vi "Call Scan Code.vi"(0 "timeout (10sec)":u32=10000 caption="超时（10秒）", 1 "baud rate (9600)":u32=9600 caption="波特率(9600)", 2 "data bits (8)":u16=8 caption="数据比特(8)" min=5 max=8 step=1, 3 "parity (0:none)":enum16{"None", "Odd", "Even", "Mark", "Space"}(ring) caption="奇偶（0:无）", 4 "写入缓冲区":string, 5 "Total Bytes":u32, 6 "Station 1":refnum<visa-resource-name>, 7 "Station 4":refnum<visa-resource-name>, 8 "Station 2":refnum<visa-resource-name>, 9 "Station 5":refnum<visa-resource-name>, 10 "Station 3":refnum<visa-resource-name>, 11 "Station 6":refnum<visa-resource-name>) -> (14 "Station 1 data":string, 15 "Station 2 data":string, 16 "Station 3 data":string, 17 "Station 4 data":string, 18 "Station 5 data":string, 19 "Station 6 data":string)   [LabVIEW 2014]
uses:
  <vilib>/Instr/_visa.llb/VISA Configure Serial Port (Instr).vi
panel:
  out "Error 6":errorcluster caption="错误输出"
  out "Error 5":errorcluster caption="错误输出"
  out "Error 4":errorcluster caption="错误输出"
  out "Error 3":errorcluster caption="错误输出"
  out "Error 2":errorcluster caption="错误输出"
  out "Error":errorcluster caption="错误输出"
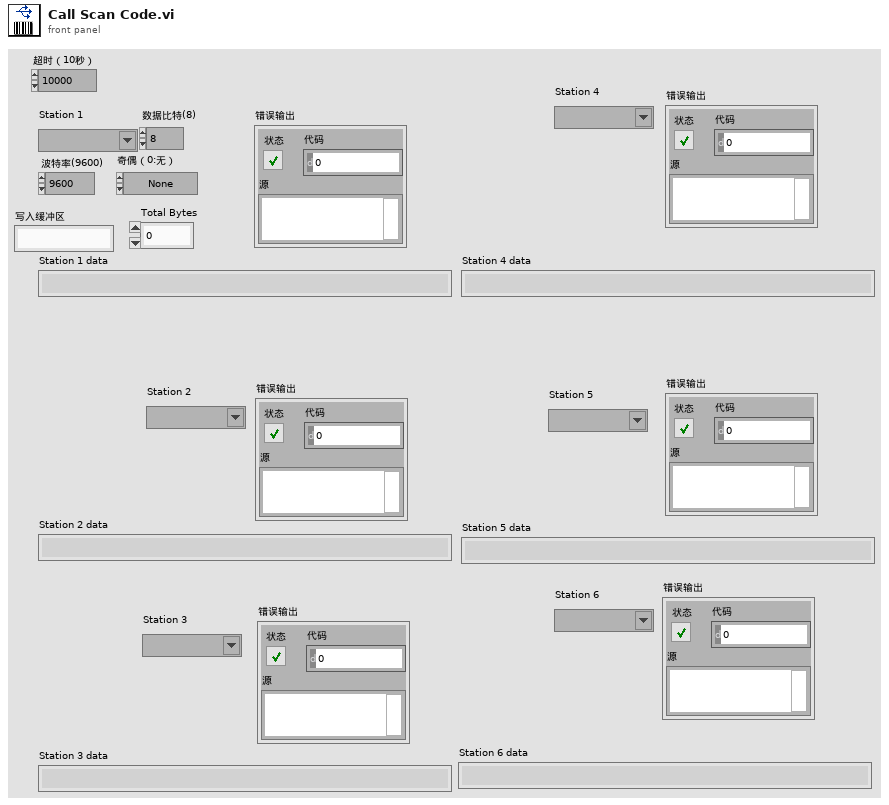
[diagram p1: front panel]
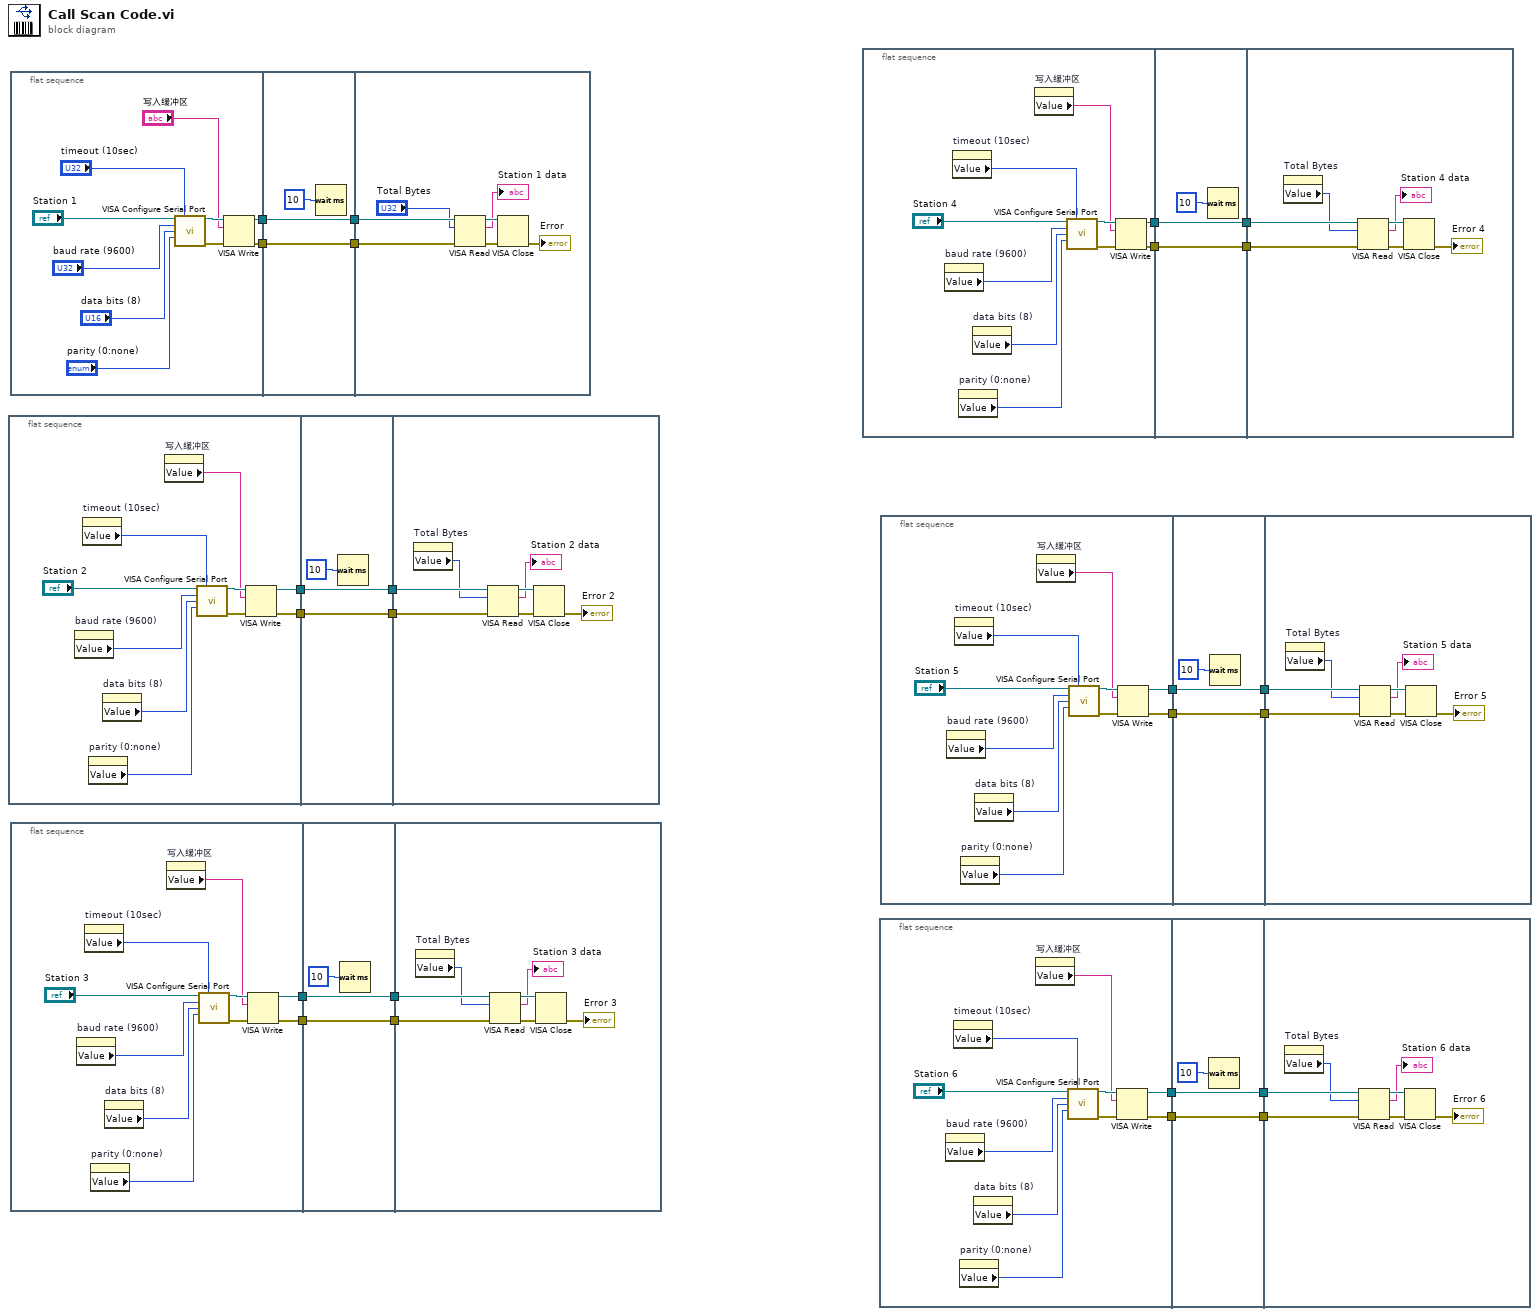
[diagram p0: block diagram]
diagram:
  n1 = flat-sequence {
    tunnel: [w31] -> w20
    tunnel: [w30] -> w19
    tunnel: [w36] -> w18
    tunnel: w20 -> [w36]
    tunnel: [w35] -> w17
    tunnel: w19 -> [w35]
    tunnel: w18 -> [w44]
    tunnel: w17 -> [w43]
    frame #0 {
      n2 = property on="baud rate (9600)" class="DigNum (严格)"() -> ("Value"=w28:u32)  [unwired: 2 in, 2 out]
      n3 = property on="timeout (10sec)" class="DigNum (严格)"() -> ("Value"=w29:u32)  [unwired: 2 in, 2 out]
      n4 = property on="parity (0:none)" class="Enum (严格)"() -> ("Value"=w26:enum16{"None", "Odd", "Even", "Mark", "Space"})  [unwired: 2 in, 2 out]
      n5 = property on="data bits (8)" class="DigNum (严格)"() -> ("Value"=w27:u16)  [unwired: 2 in, 2 out]
      n6 = property on="写入缓冲区" class="Str"() -> ("Value"=w25:string)  [unwired: 2 in, 2 out]
      n7 = call-poly "VISA Configure Serial Port"("VISA resource name"="Station 2", "timeout (10sec)"=w29, "baud rate (9600)"=w28, "data bits (8)"=w27, "parity (0:none)"=w26) -> ("VISA resource name out"=w33:refnum<visa-resource-name>, "error out"=w32:errorcluster)  [unwired: 9 in]
      n8 = VISA Write(VISA resource name=w33, write buffer=w25, error in (no error)=w32) -> (VISA resource name out=w31:refnum<visa-resource-name>, error out=w30:errorcluster)  [unwired: 1 out]
    }
    frame #1 {
      n9 = Wait (ms)(milliseconds to wait=u32 10 ("等待时间（毫秒）")) -> ()  [unwired: 1 out]
    }
    frame #2 {
      n10 = property on="Total Bytes" class="DigNum (严格)"() -> ("Value"=w38:u32)  [unwired: 2 in, 2 out]
      n11 = VISA Read(VISA resource name=w44, byte count=w38, error in (no error)=w43) -> (VISA resource name out=w42:refnum<visa-resource-name>, read buffer=→"Station 2 data":string, error out=w41:errorcluster)  [unwired: 1 out]
      n12 = VISA Close(VISA resource name=w42, error in (no error)=w41) -> (error out=→"Error 2":errorcluster)
    }
  }
  n13 = flat-sequence {
    tunnel: [w48] -> w24
    tunnel: [w47] -> w23
    tunnel: [w56] -> w22
    tunnel: w24 -> [w56]
    tunnel: [w55] -> w21
    tunnel: w23 -> [w55]
    tunnel: w22 -> [w64]
    tunnel: w21 -> [w63]
    frame #0 {
      n14 = call-poly "VISA Configure Serial Port"("VISA resource name"="Station 1", "timeout (10sec)"="timeout (10sec)", "baud rate (9600)"="baud rate (9600)", "data bits (8)"="data bits (8)", "parity (0:none)"="parity (0:none)") -> ("VISA resource name out"=w50:refnum<visa-resource-name>, "error out"=w49:errorcluster)  [unwired: 9 in]
      n15 = VISA Write(VISA resource name=w50, write buffer="写入缓冲区", error in (no error)=w49) -> (VISA resource name out=w48:refnum<visa-resource-name>, error out=w47:errorcluster)  [unwired: 1 out]
    }
    frame #1 {
      n16 = Wait (ms)(milliseconds to wait=u32 10 ("等待时间（毫秒）")) -> ()  [unwired: 1 out]
    }
    frame #2 {
      n17 = VISA Read(VISA resource name=w64, byte count="Total Bytes", error in (no error)=w63) -> (VISA resource name out=w61:refnum<visa-resource-name>, read buffer=→"Station 1 data":string, error out=w60:errorcluster)  [unwired: 1 out]
      n18 = VISA Close(VISA resource name=w61, error in (no error)=w60) -> (error out=→"Error":errorcluster)
    }
  }
  n19 = flat-sequence {
    tunnel: [w71] -> w16
    tunnel: [w70] -> w15
    tunnel: [w76] -> w14
    tunnel: w16 -> [w76]
    tunnel: [w75] -> w13
    tunnel: w15 -> [w75]
    tunnel: w14 -> [w84]
    tunnel: w13 -> [w83]
    frame #0 {
      n20 = property on="baud rate (9600)" class="DigNum (严格)"() -> ("Value"=w68:u32)  [unwired: 2 in, 2 out]
      n21 = property on="timeout (10sec)" class="DigNum (严格)"() -> ("Value"=w69:u32)  [unwired: 2 in, 2 out]
      n22 = property on="parity (0:none)" class="Enum (严格)"() -> ("Value"=w66:enum16{"None", "Odd", "Even", "Mark", "Space"})  [unwired: 2 in, 2 out]
      n23 = property on="data bits (8)" class="DigNum (严格)"() -> ("Value"=w67:u16)  [unwired: 2 in, 2 out]
      n24 = property on="写入缓冲区" class="Str"() -> ("Value"=w65:string)  [unwired: 2 in, 2 out]
      n25 = call-poly "VISA Configure Serial Port"("VISA resource name"="Station 3", "timeout (10sec)"=w69, "baud rate (9600)"=w68, "data bits (8)"=w67, "parity (0:none)"=w66) -> ("VISA resource name out"=w73:refnum<visa-resource-name>, "error out"=w72:errorcluster)  [unwired: 9 in]
      n26 = VISA Write(VISA resource name=w73, write buffer=w65, error in (no error)=w72) -> (VISA resource name out=w71:refnum<visa-resource-name>, error out=w70:errorcluster)  [unwired: 1 out]
    }
    frame #1 {
      n27 = Wait (ms)(milliseconds to wait=u32 10 ("等待时间（毫秒）")) -> ()  [unwired: 1 out]
    }
    frame #2 {
      n28 = property on="Total Bytes" class="DigNum (严格)"() -> ("Value"=w78:u32)  [unwired: 2 in, 2 out]
      n29 = VISA Read(VISA resource name=w84, byte count=w78, error in (no error)=w83) -> (VISA resource name out=w82:refnum<visa-resource-name>, read buffer=→"Station 3 data":string, error out=w81:errorcluster)  [unwired: 1 out]
      n30 = VISA Close(VISA resource name=w82, error in (no error)=w81) -> (error out=→"Error 3":errorcluster)
    }
  }
  n31 = flat-sequence {
    tunnel: [w91] -> w12
    tunnel: [w90] -> w11
    tunnel: [w96] -> w10
    tunnel: w12 -> [w96]
    tunnel: [w95] -> w9
    tunnel: w11 -> [w95]
    tunnel: w10 -> [w104]
    tunnel: w9 -> [w103]
    frame #0 {
      n32 = property on="baud rate (9600)" class="DigNum (严格)"() -> ("Value"=w88:u32)  [unwired: 2 in, 2 out]
      n33 = property on="timeout (10sec)" class="DigNum (严格)"() -> ("Value"=w89:u32)  [unwired: 2 in, 2 out]
      n34 = property on="parity (0:none)" class="Enum (严格)"() -> ("Value"=w86:enum16{"None", "Odd", "Even", "Mark", "Space"})  [unwired: 2 in, 2 out]
      n35 = property on="data bits (8)" class="DigNum (严格)"() -> ("Value"=w87:u16)  [unwired: 2 in, 2 out]
      n36 = property on="写入缓冲区" class="Str"() -> ("Value"=w85:string)  [unwired: 2 in, 2 out]
      n37 = call-poly "VISA Configure Serial Port"("VISA resource name"="Station 4", "timeout (10sec)"=w89, "baud rate (9600)"=w88, "data bits (8)"=w87, "parity (0:none)"=w86) -> ("VISA resource name out"=w93:refnum<visa-resource-name>, "error out"=w92:errorcluster)  [unwired: 9 in]
      n38 = VISA Write(VISA resource name=w93, write buffer=w85, error in (no error)=w92) -> (VISA resource name out=w91:refnum<visa-resource-name>, error out=w90:errorcluster)  [unwired: 1 out]
    }
    frame #1 {
      n39 = Wait (ms)(milliseconds to wait=u32 10 ("等待时间（毫秒）")) -> ()  [unwired: 1 out]
    }
    frame #2 {
      n40 = property on="Total Bytes" class="DigNum (严格)"() -> ("Value"=w98:u32)  [unwired: 2 in, 2 out]
      n41 = VISA Read(VISA resource name=w104, byte count=w98, error in (no error)=w103) -> (VISA resource name out=w102:refnum<visa-resource-name>, read buffer=→"Station 4 data":string, error out=w101:errorcluster)  [unwired: 1 out]
      n42 = VISA Close(VISA resource name=w102, error in (no error)=w101) -> (error out=→"Error 4":errorcluster)
    }
  }
  n43 = flat-sequence {
    tunnel: [w111] -> w4
    tunnel: [w110] -> w3
    tunnel: [w116] -> w2
    tunnel: w4 -> [w116]
    tunnel: [w115] -> w1
    tunnel: w3 -> [w115]
    tunnel: w2 -> [w124]
    tunnel: w1 -> [w123]
    frame #0 {
      n44 = property on="baud rate (9600)" class="DigNum (严格)"() -> ("Value"=w108:u32)  [unwired: 2 in, 2 out]
      n45 = property on="timeout (10sec)" class="DigNum (严格)"() -> ("Value"=w109:u32)  [unwired: 2 in, 2 out]
      n46 = property on="parity (0:none)" class="Enum (严格)"() -> ("Value"=w106:enum16{"None", "Odd", "Even", "Mark", "Space"})  [unwired: 2 in, 2 out]
      n47 = property on="data bits (8)" class="DigNum (严格)"() -> ("Value"=w107:u16)  [unwired: 2 in, 2 out]
      n48 = property on="写入缓冲区" class="Str"() -> ("Value"=w105:string)  [unwired: 2 in, 2 out]
      n49 = call-poly "VISA Configure Serial Port"("VISA resource name"="Station 6", "timeout (10sec)"=w109, "baud rate (9600)"=w108, "data bits (8)"=w107, "parity (0:none)"=w106) -> ("VISA resource name out"=w113:refnum<visa-resource-name>, "error out"=w112:errorcluster)  [unwired: 9 in]
      n50 = VISA Write(VISA resource name=w113, write buffer=w105, error in (no error)=w112) -> (VISA resource name out=w111:refnum<visa-resource-name>, error out=w110:errorcluster)  [unwired: 1 out]
    }
    frame #1 {
      n51 = Wait (ms)(milliseconds to wait=u32 10 ("等待时间（毫秒）")) -> ()  [unwired: 1 out]
    }
    frame #2 {
      n52 = property on="Total Bytes" class="DigNum (严格)"() -> ("Value"=w118:u32)  [unwired: 2 in, 2 out]
      n53 = VISA Read(VISA resource name=w124, byte count=w118, error in (no error)=w123) -> (VISA resource name out=w122:refnum<visa-resource-name>, read buffer=→"Station 6 data":string, error out=w121:errorcluster)  [unwired: 1 out]
      n54 = VISA Close(VISA resource name=w122, error in (no error)=w121) -> (error out=→"Error 6":errorcluster)
    }
  }
  n55 = flat-sequence {
    tunnel: [w131] -> w8
    tunnel: [w130] -> w7
    tunnel: [w136] -> w6
    tunnel: w8 -> [w136]
    tunnel: [w135] -> w5
    tunnel: w7 -> [w135]
    tunnel: w6 -> [w144]
    tunnel: w5 -> [w143]
    frame #0 {
      n56 = property on="baud rate (9600)" class="DigNum (严格)"() -> ("Value"=w128:u32)  [unwired: 2 in, 2 out]
      n57 = property on="timeout (10sec)" class="DigNum (严格)"() -> ("Value"=w129:u32)  [unwired: 2 in, 2 out]
      n58 = property on="parity (0:none)" class="Enum (严格)"() -> ("Value"=w126:enum16{"None", "Odd", "Even", "Mark", "Space"})  [unwired: 2 in, 2 out]
      n59 = property on="data bits (8)" class="DigNum (严格)"() -> ("Value"=w127:u16)  [unwired: 2 in, 2 out]
      n60 = property on="写入缓冲区" class="Str"() -> ("Value"=w125:string)  [unwired: 2 in, 2 out]
      n61 = call-poly "VISA Configure Serial Port"("VISA resource name"="Station 5", "timeout (10sec)"=w129, "baud rate (9600)"=w128, "data bits (8)"=w127, "parity (0:none)"=w126) -> ("VISA resource name out"=w133:refnum<visa-resource-name>, "error out"=w132:errorcluster)  [unwired: 9 in]
      n62 = VISA Write(VISA resource name=w133, write buffer=w125, error in (no error)=w132) -> (VISA resource name out=w131:refnum<visa-resource-name>, error out=w130:errorcluster)  [unwired: 1 out]
    }
    frame #1 {
      n63 = Wait (ms)(milliseconds to wait=u32 10 ("等待时间（毫秒）")) -> ()  [unwired: 1 out]
    }
    frame #2 {
      n64 = property on="Total Bytes" class="DigNum (严格)"() -> ("Value"=w138:u32)  [unwired: 2 in, 2 out]
      n65 = VISA Read(VISA resource name=w144, byte count=w138, error in (no error)=w143) -> (VISA resource name out=w142:refnum<visa-resource-name>, read buffer=→"Station 5 data":string, error out=w141:errorcluster)  [unwired: 1 out]
      n66 = VISA Close(VISA resource name=w142, error in (no error)=w141) -> (error out=→"Error 5":errorcluster)
    }
  }
